vi "ReadDispParams.vi"() -> ()   [LabVIEW 2015]
uses:
  GlobalDisplayIndex.vi
panel:
  out "Array":i32[](array[numeric])
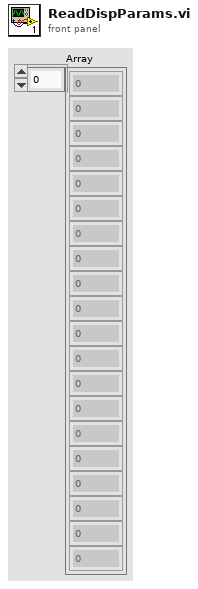
[diagram p1: front panel]
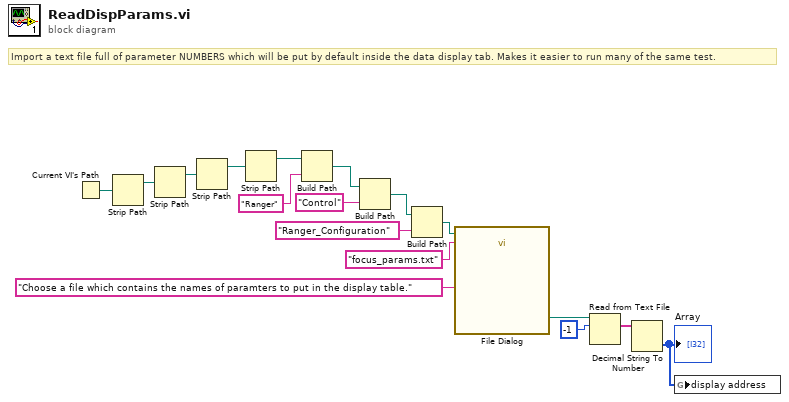
[diagram p0: block diagram]
diagram:
  # "Import a text file full of parameter NUMBERS which will be put by default inside the data display tab. Makes it easier to run many of the same test."
  n1 = Current VI's Path() -> (path=w11:path)
  n2 = Strip Path(path=w11) -> (stripped path=w10:path)  [unwired: 1 out]
  n3 = Strip Path(path=w10) -> (stripped path=w9:path)  [unwired: 1 out]
  n4 = Strip Path(path=w9) -> (stripped path=w8:path)  [unwired: 1 out]
  n5 = Strip Path(path=w8) -> (stripped path=w7:path)  [unwired: 1 out]
  n6 = Build Path(base path=w7, name or relative path="Ranger") -> (appended path=w6:path)
  n7 = Build Path(base path=w6, name or relative path="Control") -> (appended path=w3:path)
  n8 = Build Path(base path=w3, name or relative path="Ranger_Configuration") -> (appended path=w2:path)
  n9 = call "File Dialog"("start path"=w2, "prompt"="Choose a file which contains the names of paramters to put in the display table.", "default name"="focus_params.txt" ("name or relative path")) -> ("selected path"=w15:path)  [unwired: 9 in, 3 out]
  n10 = Read from Text File(file (use dialog)=w15, count=-1) -> (text=w13:string[])  [unwired: 2 in, 3 out]
  n11 = Decimal String To Number(string=w13) -> (number=w1:i32[])  [unwired: 2 in, 1 out]
  "Array" <- w1
  n12 = global write "GlobalDisplayIndex.vi" "display address"(w1) -> ()
